vi "TestRegisterVI.vi"(8 "error in (no error)":errorcluster) -> (0 "error out":errorcluster)   [LabVIEW 2017]
uses:
  src/Private/RegisterVI.vi
  <vilib>/addons/_JKI Toolkits/Caraya/classes/Test/Test.lvclass
  src/API/JKI Simple Localization.lvlib
  <vilib>/addons/_JKI Toolkits/Caraya/classes/Assert/Assert.lvclass
panel:
  # "See block diagram for unit tests of RegisterVI.vi"
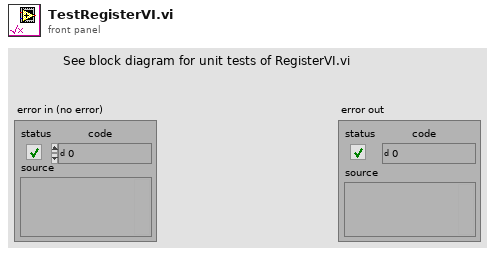
[diagram p1: front panel]
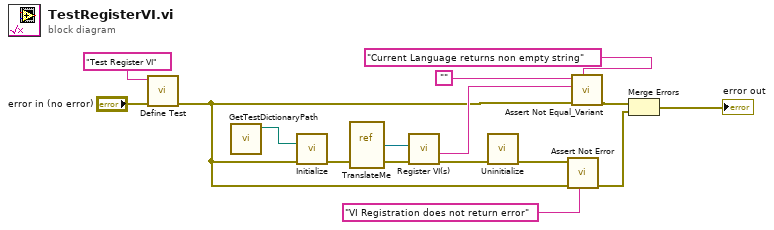
[diagram p0: block diagram]
diagram:
  n1 = call <vilib>:"Define Test.vi"("error in (no error)"="error in (no error)", "Label (VI Title)"="Test Register VI") -> ("error out"=w4:errorcluster)  [unwired: 9 in]
  n2 = call "GetTestDictionaryPath.vi"() -> ("Test Dictionary Path"=w12:path)  [unwired: 11 in]
  n3 = call "Initialize.vi"("Dictionary File Path"=w12, "error in"=w4) -> ("error out"=w11:errorcluster)  [unwired: 10 in, 3 out]
  n4 = vi-ref "TranslateMe.vi"() -> (w13:refnum<vi>)
  n5 = call-poly "Register VI(s).vi"("error in"=w11, "VI Ref"=w13) -> ("error out"=w5:errorcluster, "Current Language"=w7:string)  [unwired: 8 in]
  n6 = call "Uninitialize.vi"("error in"=w5) -> ("error out"=w1:errorcluster)  [unwired: 10 in]
  n7 = call <vilib>:"Assert Not Error.vi"("Label"="VI Registration does not return error", "error in (no error)"=w4, "Not Error?"=w1) -> ("error out"=w3:errorcluster)  [unwired: 8 in]
  n8 = call <vilib>:"Assert Not Equal_Variant.vi"("Label"="Current Language returns non empty string", "error in (no error)"=w4, "Y"=w7, "X"="") -> ("error out"=w9:errorcluster)  [unwired: 7 in]
  n9 = Merge Errors(w9, w3) -> (→"error out":errorcluster)
